vi "Find_Default_Gateway.vi"(8 "Error In":errorcluster) -> (0 "Error Out":errorcluster, 3 "Default Gateway":string)   [LabVIEW 2017]
panel:
  out "Terminal Output":string
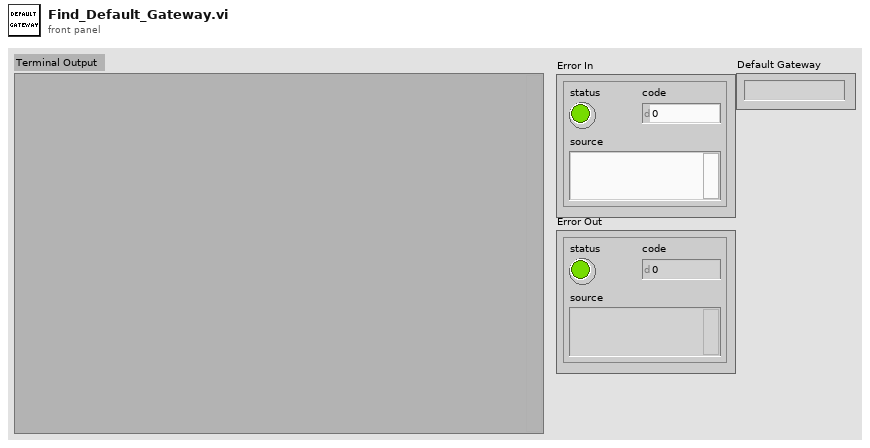
[diagram p1: front panel]
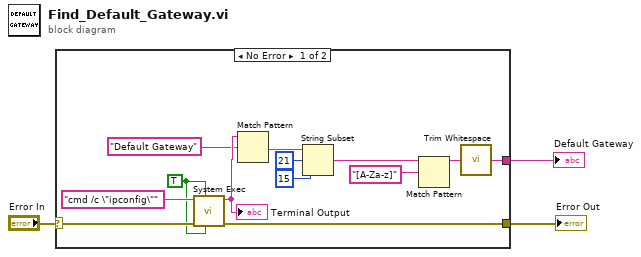
[diagram p0: block diagram]
diagram:
  n1 = case shown="No Error" "Error In" {
    selector: "Error In" -> [w14 w17]
    tunnel: [w4 _] -> w1
    tunnel: [w13 w17] -> w2
    frame No Error {
      w8 = TRUE ("wait until completion? (T)")
      n2 = call <vilib>:"System Exec.vi"("run minimized? (F)"=w8, "wait until completion? (T)"=w8, "error in (no error)"=w14, "command line"="cmd /c \"ipconfig\"") -> ("error out"=w13:errorcluster, "standard output"=w16:string)  [unwired: 4 in, 2 out]
      "Terminal Output" <- w16
      n3 = Match Pattern(string=w16, regular expression="Default Gateway") -> (after substring=w11:string)  [unwired: 1 in, 3 out]
      n4 = String Subset(string=w11, offset (0)=21, length (rest)=15 ("length (rest)")) -> (substring=w6:string)
      n5 = Match Pattern(string=w6, regular expression="[A-Za-z]") -> (before substring=w5:string)  [unwired: 1 in, 3 out]
      n6 = call <vilib>:"Trim Whitespace.vi"("string"=w5) -> ("trimmed string"=w4:string)  [unwired: 1 in]
    }
    frame Error {
    }
  }
  "Error Out" <- w2
  "Default Gateway" <- w1
